vi "Test Report Generation.vi"(8 "error in (no error)":errorcluster) -> (0 "error out":errorcluster, 3 "Succeeded?":bool)   [LabVIEW 2013]
uses:
  classes/Test Suite/Test Suite.lvclass
  classes/Test Suite/Define Test Suite (SimpleText Report).vi
panel:
  out "Test Report File Contents":string
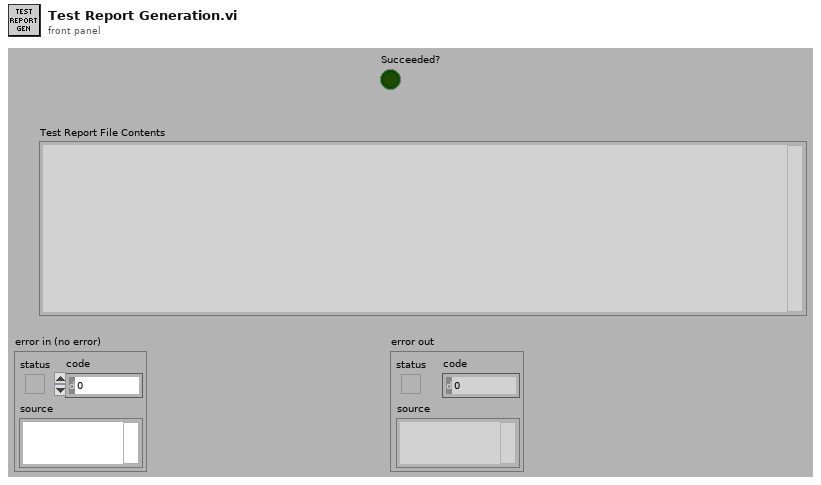
[diagram p1: front panel]
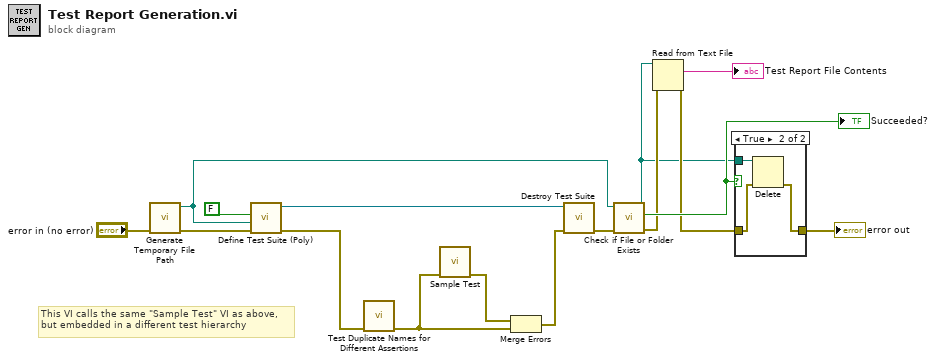
[diagram p0: block diagram]
diagram:
  # "This VI calls the same \"Sample Test\" VI as above,\nbut embedded in a different test hierarchy"
  n1 = call <vilib>:"Generate Temporary File Path.vi"("error in (no error)"="error in (no error)") -> ("error out"=w6:errorcluster, "Unique Temporary File Path"=w5:path)  [unwired: 9 in]
  n2 = call-poly "Define Test Suite (Poly).vi"("error in (no error)"=w6, "Report Path"=w5, "Interactive"=FALSE) -> ("error out"=w2:errorcluster, "Test Suite"=w7:refnum<class "Test Suite.lvclass">)  [unwired: 7 in]
  n3 = call "Test Duplicate Names for Different Assertions.vi"("error in (no error)"=w2) -> ("error out"=w1:errorcluster)  [unwired: 10 in]
  n4 = call "Sample Test.vi"("error in (no error)"=w1) -> ("error out"=w3:errorcluster)  [unwired: 10 in]
  n5 = Merge Errors(w3, w1) -> (w4:errorcluster)
  n6 = call-dynamic "Destroy Test Suite.vi"("error in (no error)"=w4, "Test Suite in"=w7) -> ("error out"=w15:errorcluster)  [unwired: 9 in]
  n7 = call <vilib>:"Check if File or Folder Exists.vi"("error in (no error)"=w15, "path"=w5) -> ("error out"=w12:errorcluster, "file or folder exists?"=w14:bool, "dup path"=w9:path)  [unwired: 7 in]
  "Succeeded?" <- w14
  n8 = Read from Text File(file (use dialog)=w9, error in=w12) -> (text=→"Test Report File Contents":string, error out=w11:errorcluster)  [unwired: 2 in, 2 out]
  n9 = case shown="True" w14 {
    tunnel: w9 -> [_ w20]
    tunnel: w11 -> [w17 w19]
    tunnel: [w17 w18] -> w13
    frame False {
    }
    frame True {
      n10 = Delete(path (use dialog)=w20, error in=w19) -> (error out=w18:errorcluster)  [unwired: 3 in, 2 out]
    }
  }
  "error out" <- w13
